vi "Update SubComponent Data (EXT).vi"(8 "error in (no error)":errorcluster, 9 "Data":u16[](array[numeric]), 10 "Addresses":u16[](array[numeric]), 11 "1553 SubComponent in":refnum<class "1553 SubComponent.lvclass">) -> (0 "error out":errorcluster, 3 "1553 SubComponent out":refnum<class "1553 SubComponent.lvclass">)   [LabVIEW 2020, in "BCI-1553 API.lvlib" / "1553 SubComponent.lvclass"]
doc: "<UNIMPLEMENTED>\n\nProvides a means for handling externally-retrieved data values. The supplied address list must be cross-referenced with a configured parameter and the data value(s) should be stored with that parameter as the current value.\n\nUnused addresses are ignored and unmodified parameters shall retain their prior value."
uses:
  1553 SubComponent.lvclass
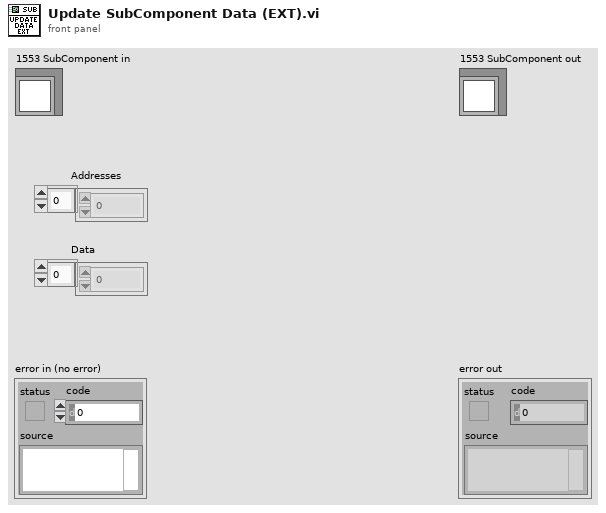
[diagram p1: front panel]
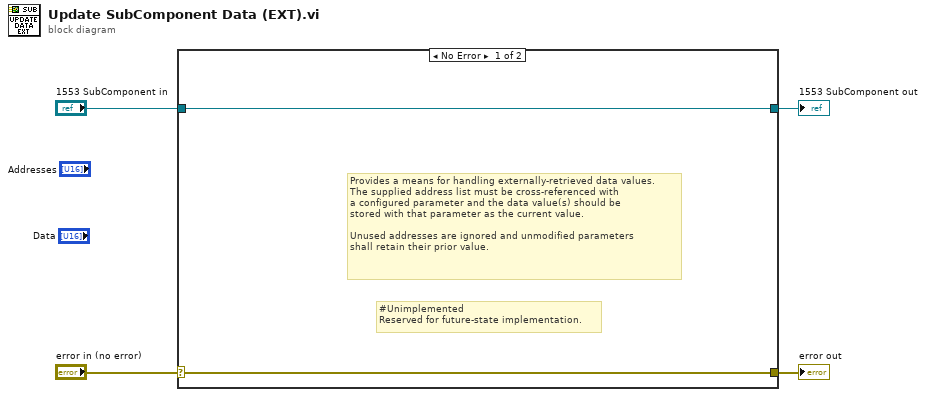
[diagram p0: block diagram]
diagram:
  n1 = case shown="No Error" "error in (no error)" {
    selector: "error in (no error)" -> [w5 w8]
    tunnel: [w5 w8] -> w3
    tunnel: [w6 w7] -> w1
    tunnel: "1553 SubComponent in" -> [w6 w7]
    frame No Error {
      # "#Unimplemented\nReserved for future-state implementation."
      # "Provides a means for handling externally-retrieved data values.\nThe supplied address list must be cross-referenced with\na configured parameter and the data value(s) should be\nstored with that parameter as the current value.\n\nUnused addresses are ignored and unmodified parameters\nshall retain their prior value."
    }
    frame Error {
    }
  }
  "error out" <- w3
  "1553 SubComponent out" <- w1
